vi "Add Event Record.vi"(10 "event tag":string, 11 "event records in":string[](array[string])) -> (3 "event records out":string[](array[string]))   [LabVIEW 2021, in "Game of Life.lvlib"]
doc: "Appends the provided 'Event tag' and current Date -Time string to the provided 'Event Records' array."
uses:
  Game of Life.lvlib
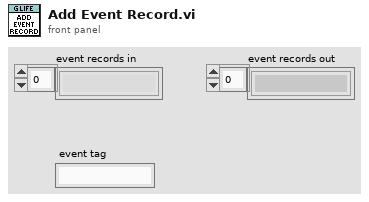
[diagram p1: front panel]
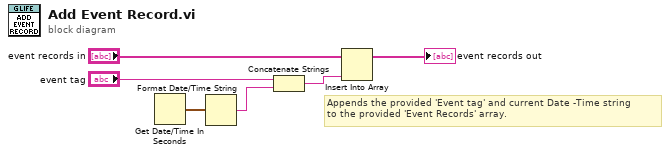
[diagram p0: block diagram]
diagram:
  # "Appends the provided 'Event tag' and current Date -Time string\nto the provided 'Event Records' array."
  n1 = Get Date/Time In Seconds() -> (seconds since 1Jan1904=w4:timestamp)
  n2 = Format Date/Time String(seconds (now)=w4) -> (date/time string=w2:string)  [unwired: 2 in]
  n3 = Concatenate Strings("event tag", w2) -> (w3:string)
  n4 = Insert Into Array(array="event records in", new element=w3) -> (→"event records out":string[])  [unwired: 1 in]
